vi "LS_DAQ_RealTime.vi"() -> ()   [LabVIEW 2020]
uses:
  <vilib>/Platform/TimedLoop/XDataNode/timing_clust.ctl
  <vilib>/Platform/TimedLoop/XDataNode/nitl_modes.ctl
  <vilib>/Platform/TimedLoop/XDataNode/wakeup.ctl
  <vilib>/platform/TimedLoop/XDataNode/XDataNode.xnode
  <vilib>/Platform/TimedLoop/XDataNode/XDNodeRunTimeDep.lvlib
panel:
  out "Pulse count":dbl
  out "Period [ms]":u32
  out "Data":dbl[](array[numeric])
  out "error IO":errorcluster
  out "Finished Late? [i-1]":bool
  out "Iteration Duration":i64
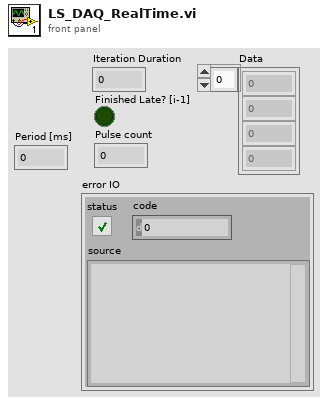
[diagram p1: front panel]
types:
  T1 = typedef "XDNodeRunTimeDep.lvlib/timing_clust.ctl" = cluster{"Expected End [f-1]":u64, "Actual End [f-1]":u64, "Finished Late? [f-1]":bool, "Expected End [i-1]":u64, "Actual End [i-1]":u64, "Finished Late? [i-1]":bool, "Expected Start [i]":u64, "Actual Start [i]":u64, "Expected Start [f]":u64, "Actual Start [f]":u64, "Source Name":string, "Structure Name":string, "Period":i64, "Deadline":i64, "Offset":i64, "Start":i64, "Priority":i32, "Timeout":i32, "Mode":T2, "Wakeup Reason":T3, "Error":errorcluster, "Source Type":string, "Secondary Source Type":string, "Global End Time":u64, "Global Start Time":u64, "Frame Duration":u64, "Iteration Duration":u64, "Assigned CPU":i32, "I/O Scan Engine Mode":u32}
  T2 = typedef "XDNodeRunTimeDep.lvlib/nitl_modes.ctl" = enum32{"No Change", "Process missed periods, maintain original phase", "Discard missed periods, maintain original phase", "Process missed periods, ignore original phase", "Discard missed periods, ignore original phase"}
  T3 = typedef "XDNodeRunTimeDep.lvlib/wakeup.ctl" = enum32{"Normal", "Aborted", "Asynchronous wakeup", "Timing source error", "Timed loop error", "Timeout"}
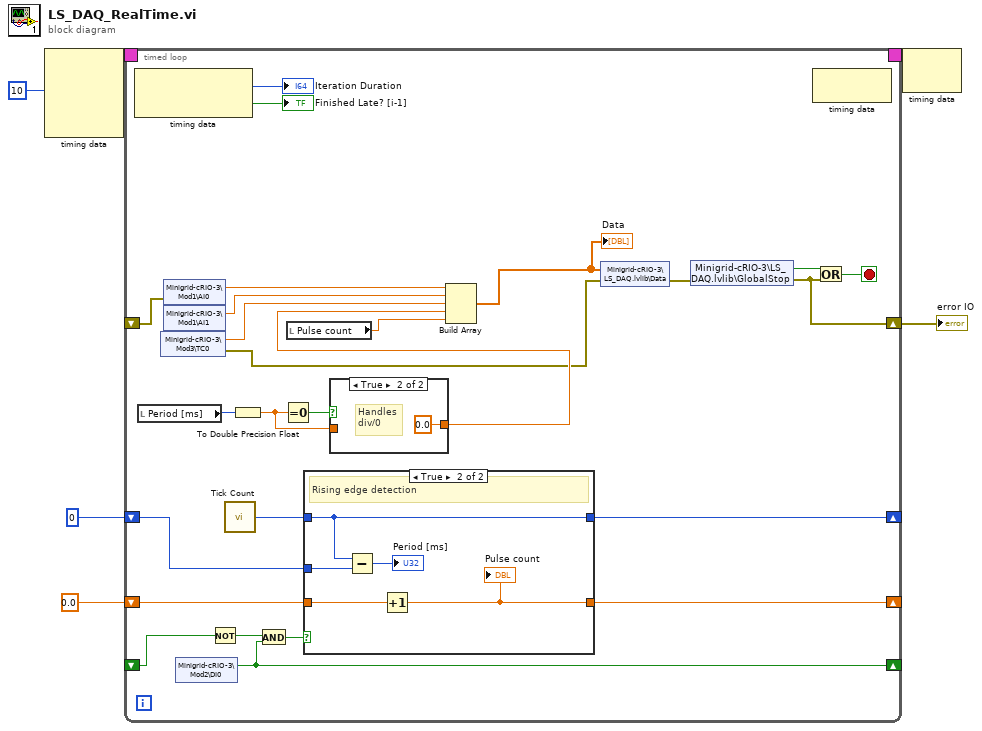
[diagram p0: block diagram]
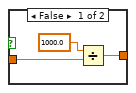
[diagram p2: hidden frame]
diagram:
  n1 = node-c288(i64 10 ("Period")) -> (w6:T1)  [unwired: 3 in]
  n2 = timed-loop {
    timing: w6 -> [_]
    timing-out: [_] -> w5
    shift-right: [w18] -> w1
    shift-left: _ -> [w30]
    shift-right: [w14] -> _
    shift-left: u32 0 ("Tick Count(uSec)") -> [w25]
    shift-right: [w24] -> _
    shift-left: _ -> [w23]
    shift-right: [w21] -> _
    shift-left: 0.0 ("Tick Count(uSec)") -> [w22]
    stop <- w20 stop-if-true
    n3 = node-c288() -> (→"Iteration Duration":i64, →"Finished Late? [i-1]":bool)  [unwired: 1 in]
    n4 = local read "Period [ms]"() -> (w17:u32)
    n5 = shared-variable "Minigrid-cRIO-3\\Mod1\\AI0"(error in=w30) -> (w32:dbl, error out=w29:errorcluster)
    n6 = shared-variable "Minigrid-cRIO-3\\Mod1\\AI1"(error in=w29) -> (w31:dbl, error out=w8:errorcluster)
    n7 = shared-variable "Minigrid-cRIO-3\\Mod3\\TC0"(error in=w8) -> (w9:dbl, error out=w7:errorcluster)
    n8 = shared-variable "Minigrid-cRIO-3\\Mod2\\DI0"() -> (w24:bool)  [unwired: 1 in, 1 out]
    n9 = Not(x=w23) -> (.not. x?=w28:bool)
    n10 = call "Tick Count"() -> ("Tick Count(mSec)"=w26:u32)
    n11 = To Double Precision Float(number=w17) -> (double precision float=w15:dbl)
    n12 = And(x=w28, y=w24) -> (x .and. y?=w27:bool)
    n13 = Equal To 0?(x=w15) -> (x = 0?=w16:bool)
    n14 = local read "Pulse count"() -> (w11:dbl)
    n15 = case shown="True" w27 {
      tunnel: w26 -> [_ w41]
      tunnel: w25 -> [w39 w45]
      tunnel: w22 -> [w40 w43]
      tunnel: [w40 w42] -> w21
      tunnel: [w39 w41] -> w14
      frame False {
      }
      frame True {
        # "Rising edge detection"
        n16 = Subtract(x=w41, y=w45) -> (x-y=→"Period [ms]":u32)
        n17 = Increment(x=w43) -> (x+1=w42:dbl)
        "Pulse count" <- w42
      }
    }
    n18 = case shown="True" w16 {
      tunnel: w15 -> [w37 _]
      tunnel: [w35 0.0] -> w10
      frame False {
        n19 = Divide(x=1000.0, y=w37) -> (x/y=w35:dbl)
      }
      frame True {
        # "Handles\ndiv/0"
      }
    }
    n20 = Build Array(w32, w31, w9, w10, w11) -> (w13:dbl[])
    "Data" <- w13
    n21 = shared-variable "Minigrid-cRIO-3\\LS_DAQ.lvlib\\Data"(w13, error in=w7) -> (error out=w12:errorcluster)
    n22 = shared-variable "Minigrid-cRIO-3\\LS_DAQ.lvlib\\GlobalStop"(error in=w12) -> (w19:bool, error out=w18:errorcluster)
    n23 = node-c288() -> ()  [unwired: 1 in, 1 out]
    n24 = Or(x=w19, y=w18) -> (x .or. y?=w20:bool)
  }
  "error IO" <- w1
  n25 = node-c288(w5) -> ()  [unwired: 1 out]
